vi "Dashboard Main.vi"() -> ()   [LabVIEW 2013]
uses:
  <vilib>/event_ctls.llb/eventvkey.ctl
  <vilib>/Rock Robotics/WPI/Dashboard/WPI_DashboardLogging Global.vi
  <vilib>/Utility/config.llb/Write Key (String).vi
  <vilib>/Utility/config.llb/Write Key (I32).vi
  <vilib>/Utility/config.llb/NI_LVConfig.lvlib
panel:
  out "Image Message":string="Timeout in Camera Communications"
  in  "Rec Mode":enum32{"Stop", "Record", "Playback"}(radio)
  in  "Dashboard Tab":T1(tab)
  out "Ultrasonic Sensor":dbl
  in  "Camera Settings":T2={"Frame Rate"=30, "Compression"=30, "Size"=1} {"Frame Rate" scale=1.0..30.0; "Size" items=["640x480", "320x240", "160x120"]}
  out "MotorSliders R":cluster{"MotorSlide1":dbl, "MotorSlide2":dbl} {"MotorSlide2" scale=-1.0..1.0 scale format="%#_2e"; "MotorSlide1" scale=-1.0..1.0 scale format="%#_2e"}
  out "MotorChart R":cluster{"Numeric":dbl, "Numeric":dbl}(graph)
  out "MotorSliders L":T3 {"MotorSlide4 2" scale=0.0..14.0 scale format="%#_2e"; "MotorSlide2" scale=-1.0..1.0 scale format="%#_2e"; "MotorSlide1" scale=-1.0..1.0 scale format="%#_2e"}
  out "MotorChart L":T4(graph)
  out "JS1 Z":dbl(slide) scale=-1.0..1.0 scale format="%#_2e"
  out "Joystick 1":cluster{"X":dbl, "Y":dbl}[](graph)
  out "JS Buttons 1":T5
  out "JS2 Z":dbl(slide) scale=-1.0..1.0 scale format="%#_2e"
  out "Joystick 2":cluster{"X":dbl, "Y":dbl}[](graph)
  out "JS Buttons 2":T5
  out "Mode":T6(ring)=enum."Auto Disabled"
  out "Camera IP":string
  in  "DB Camera Config":bool
  out "fps":dbl format="%#.1g"
  out "Mbps":dbl format="%#.1g"
  out "Mbps 2":bool
  out "LED 1":bool
  out "String POT":dbl
  in  "Slider 1":dbl(slide) scale=0.0..100.0
  in  "Checkbox 2":bool
  in  "Checkbox 1":bool
  in  "Test Slider":dbl(slide) scale=0.0..100.0 scale format="%#_3g"
  in  "On/Off":bool caption="Solenoid"
  in  "Test Name":u16(ring) items=["Select the test to run...", "Example Test", "-------------------------------", "List of tests is built in robot code.", "Replace with your own automated tests."]
  in  "Test Tree":string(tree)
  in  "Motor":cluster{"Value":dbl, "Enable":bool} {"Value" scale=-1.0..1.0 scale format="%#_3g"}
  out "Progress":T7 {"Test Progress" scale=0.0..100.0}
  in  "Rev/Fwd":cluster{"Forward":bool, "Reverse":bool}
  in  "Test Ring":u16(ring) items=["Auto", "Fixed indoor", "Fixed outdoor 1", "Fixed outdoor 2", "Fixed fluorescent 1", "Fixed fluorescent 2", "Hold current"]
  in  "Listbox":i32(listbox)
  out "Tree":string(tree)
  out "Camera Image":T8(plugin-control)
  in  "Enable":bool
  # "Left"
  # "Front"
  # "Right"
  # "Battery"
  # "Customize by placing controls and indicators here and name to\nmatch Dashboard Variables on robot."
  # "This tab is a great place for autonomous settings and validation.\nCustomize by placing controls and indicators here and name to\nmatch Dashboard Variables on robot."
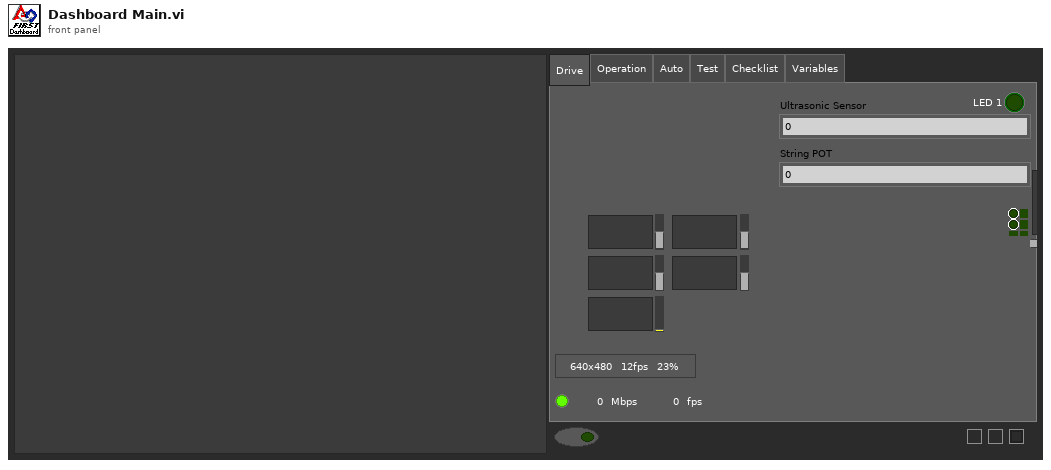
[diagram p1: front panel]
types:
  T1 = enum32{"Drive", "Operation", "Auto", "Test", "Checklist", "Variables"}
  T2 = cluster{"Frame Rate":i32, "Compression":i32, "Size":u16}
  T3 = cluster{"MotorSlide1":dbl, "MotorSlide2":dbl, "MotorSlide4 2":dbl}
  T4 = cluster{"Numeric":dbl, "Numeric":dbl, "Battery":sgl}
  T5 = cluster{bool, bool, bool, bool, bool, bool, bool, bool, bool, bool, bool, bool}
  T6 = enum8{"Tele-Op Disabled", "Tele-Op Enabled", "Auto Disabled", "Auto Enabled", "Test Disabled", "Test Enabled", ""}
  T7 = cluster{"Test Progress":u8, "Test Progress Text":string}
  T8 = typedef "IMAQ Image.ctl" = refnum<image>
  T9 = typedef "Image Type" = u32
  T10 = cluster{"Digital Inputs":bool[], "Digital Outputs":bool[]}
  T11 = cluster{"Competition mode":bool, "Robot Link":bool, "Autonomous":bool, "Enabled":bool, "E-Stop":bool, "Simulated":bool, "TestMode":bool, "Docked Window":bool}
  T12 = cluster{"Boolean Array[0]":bool, "Boolean Array[1]":bool, "Boolean Array[2]":bool, "Boolean Array[3]":bool, "Boolean Array[4]":bool, "Boolean Array[5]":bool, "Boolean Array[6]":bool, "Boolean Array[7]":bool, "Boolean Array[8]":bool, "Boolean Array[9]":bool, "Boolean Array[10]":bool, "Boolean Array[11]":bool}
  T13 = typedef "NI_LVConfig.lvlib/Config Data RefNum.ctl" = refnum<k1>
  T14 = typedef "eventvkey.ctl" = enum16{"ASCII", "Enter", "Return", "Shift", "Ctrl", "Alt", "Cmd", "Opt", "Caps", "NumLock", "Clear", "Break", "Up", "Down", "Left", "Right", "Insert", "Delete", "Home", "End", "PageUp", "PageDown", "Escape", "Help", "Pause", "ScrollLock", "F1", "F2", "F3", "F4", "F5", "F6", "F7", "F8", "F9", "F10", "F11", "F12", "F13", "F14", "F15", "F16", "F17", "F18", "F19", "F20", "F21", "F22", "F23", "F24", "Play", "VolumeUp", "VolumeDown", "Mute", "Two Byte Char"}
  T15 = cluster{"Image Size":bool, "Image Type":bool, "Pixel Value":bool, "ROI Information":bool, "Zoom Factor":bool}
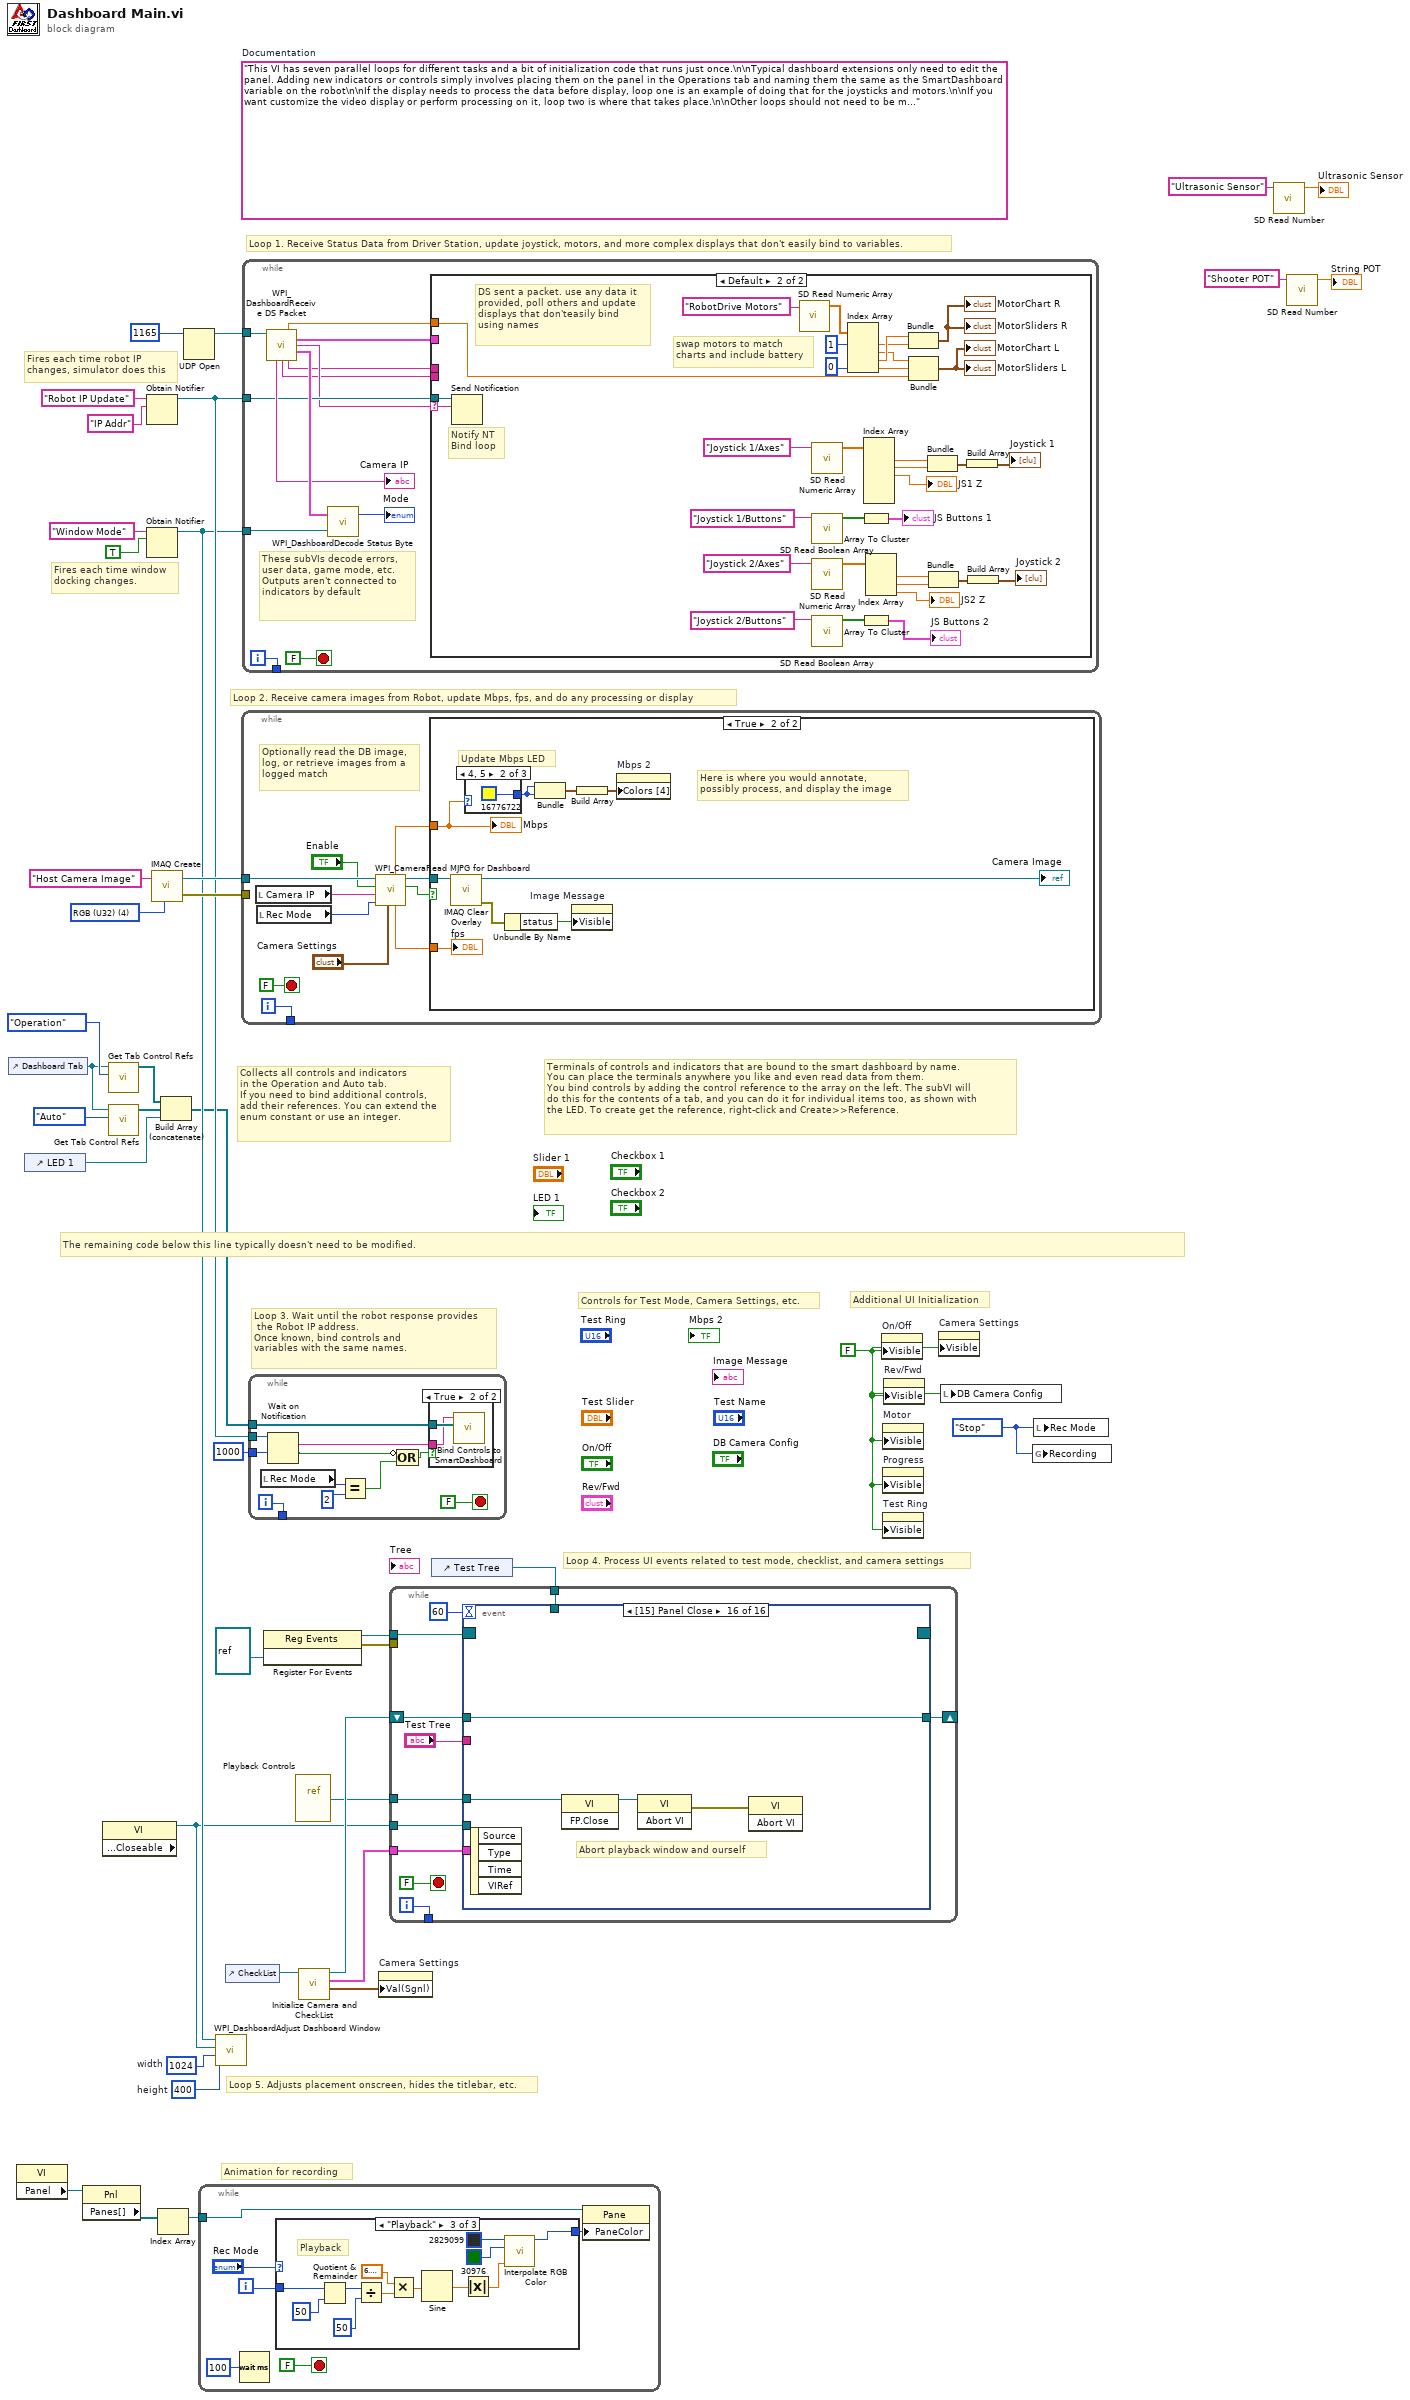
[diagram p0: block diagram]
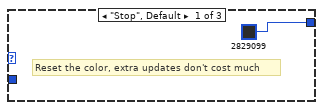
[diagram p2: hidden frame]
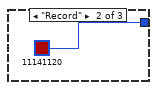
[diagram p3: hidden frame]
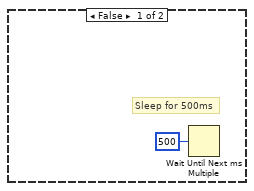
[diagram p5: hidden frame]
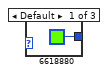
[diagram p6: hidden frame]
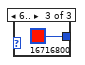
[diagram p7: hidden frame]
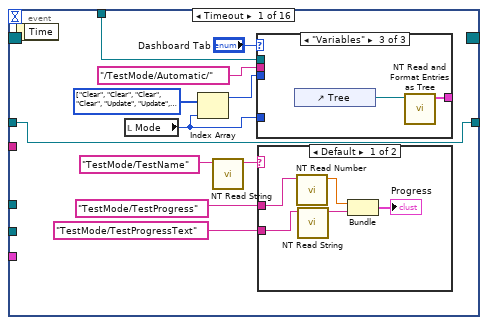
[diagram p8: hidden frame]
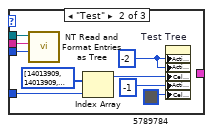
[diagram p10: hidden frame]
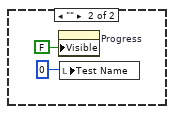
[diagram p11: hidden frame]
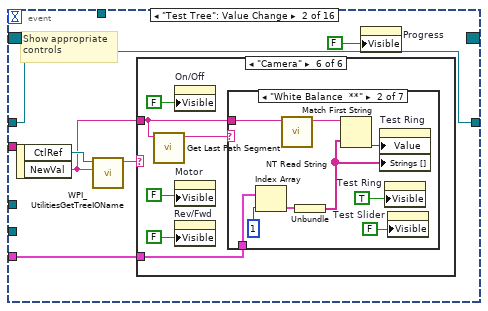
[diagram p12: hidden frame]
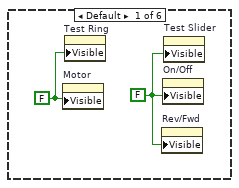
[diagram p13: hidden frame]
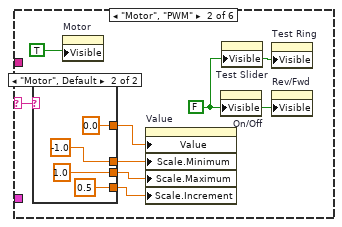
[diagram p14: hidden frame]
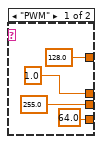
[diagram p15: hidden frame]
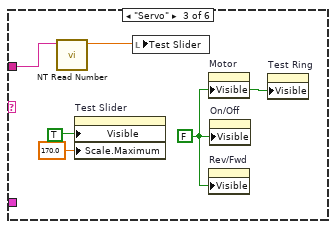
[diagram p16: hidden frame]
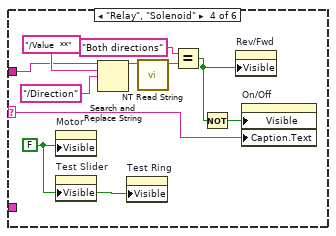
[diagram p17: hidden frame]
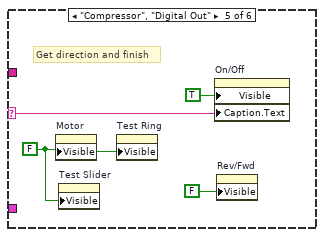
[diagram p18: hidden frame]
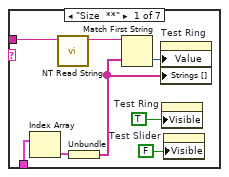
[diagram p19: hidden frame]
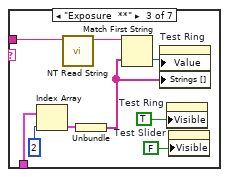
[diagram p20: hidden frame]
diagram:
  w12 = enum32{"Stop", "Record", "Playback"}."Stop" ("Rec Mode")
  w15 = 400  # height
  w16 = 1024  # width
  w29 = FALSE ("Visible")
  (unwired) "This VI has seven parallel loops for different tasks and a bit of initialization code that runs just once.\n\nTypical dashboard extensions only need to edit the panel. Adding new indicators or controls simply involves placing them on the panel in the Operations tab and naming them the same as the SmartDashboard variable on the robot\n\nIf the display needs to process the data before display, loop one is an example of doing that for the joysticks and motors.\n\nIf you want customize the video display or perform processing on it, loop two is where that takes place.\n\nOther loops should not need to be modified. They are pretty standard, and document the task they perform."  # Documentation
  w39 = T9 4 items=["Grayscale (U8)", "Grayscale (I16)", "Grayscale (SGL)", "Complex (CSG)", "RGB (U32)", "HSL (U32)", "RGB (U64)"] ("Image Type")
  # "Controls for Test Mode, Camera Settings, etc."
  # "Additional UI Initialization"
  # "Animation for recording"
  # "Fires each time robot IP\nchanges, simulator does this"
  # "Fires each time window\ndocking changes."
  # "Collects all controls and indicators\nin the Operation and Auto tab.\nIf you need to bind additional controls,\nadd their references. You can extend the\nenum constant or use an integer."
  # "The remaining code below this line typically doesn't need to be modified."
  # "Loop 4. Process UI events related to test mode, checklist, and camera settings"
  # "Terminals of controls and indicators that are bound to the smart dashboard by name.\nYou can place the terminals anywhere you like and even read data from them.\nYou bind controls by adding the control reference to the array on the left. The subVI will\ndo this for the contents of a tab, and you can do it for individual items too, as shown with\nthe LED. To create get the reference, right-click and Create>>Reference."
  # "Loop 3. Wait until the robot response provides\n the Robot IP address.\nOnce known, bind controls and\nvariables with the same names."
  # "Loop 5. Adjusts placement onscreen, hides the titlebar, etc."
  # "Loop 1. Receive Status Data from Driver Station, update joystick, motors, and more complex displays that don't easily bind to variables."
  # "Loop 2. Receive camera images from Robot, update Mbps, fps, and do any processing or display"
  n1 = control-ref of="Dashboard Tab"() -> (w10:refnum<vi>)
  n2 = property class="VI"() -> ("Panel"=w23:refnum<vi>)  [unwired: 2 in, 2 out]
  n3 = control-ref of="LED 1"() -> (w5:refnum<vi>)
  n4 = property class="Pnl"(reference=w23) -> ("Panes[]"=w24:refnum<vi>[])  [unwired: 1 in, 2 out]
  n5 = property class="VI" props=["Front Panel.Closeable"]() -> (reference out=w11:refnum<vi>)  [unwired: 2 in, 2 out]
  n6 = call <vilib>:"Get Tab Control Refs.vi"("Page Index"=T1."Operation" ("Dashboard Tab"), "TabControl in"=w10) -> ("ControlsOnPage"=w8:refnum<vi>[])  [unwired: 9 in]
  n7 = call <vilib>:"Get Tab Control Refs.vi"("Page Index"=T1."Auto" ("Dashboard Tab"), "TabControl in"=w10) -> ("ControlsOnPage"=w9:refnum<vi>[])  [unwired: 9 in]
  n8 = Obtain Notifier(name (unnamed)="Robot IP Update", notification data type="IP Addr" ("name (unnamed)")) -> (notifier out=w33:refnum<notifier>)  [unwired: 2 in, 2 out]
  n9 = Obtain Notifier(name (unnamed)="Window Mode", notification data type=TRUE) -> (notifier out=w14:refnum<notifier>)  [unwired: 2 in, 2 out]
  n10 = call "IMAQ Create"("Image Name"="Host Camera Image", "Image Type"=w39) -> ("New Image"=w37:T8, "error out"=w36:errorcluster)  [unwired: 2 in, 1 out]
  n11 = Index Array(array=w24) -> (element=w22:refnum<vi>)  [unwired: 1 in]
  n12 = Build Array (concatenate)(w8, w9, w5) -> (w7:refnum<vi>[])
  n13 = UDP Open(11:u16 1165 ("port")) -> (port=w40:refnum<k16>)  [unwired: 2 in, 4 out]
  n14 = while {
    tunnel: w22 -> [w43]
    i -> [w46]
    stop <- FALSE stop-if-true
    n15 = Wait (ms)(milliseconds to wait=u32 100) -> ()  [unwired: 1 out]
    n16 = case shown="\"Playback\"" "Rec Mode" {
      tunnel: w46 -> [_ _ w61]
      tunnel: [u32 2829099 ("Base Color") u32 11141120 ("Target Color") w50] -> w42
      frame "Stop", Default {
        # "Reset the color, extra updates don't cost much"
      }
      frame "Record" {
      }
      frame "Playback" {
        # "Playback"
        n17 = Quotient & Remainder(x=w61, y=u32 50 ("milliseconds to wait")) -> (x-y*floor(x/y)=w57:u32)  [unwired: 1 out]
        n18 = Divide(x=w57, y=u32 50 ("milliseconds to wait")) -> (x/y=w54:dbl)
        n19 = Multiply(x=6.283185307179586, y=w54) -> (x*y=w59:dbl)
        n20 = Sine(x=w59) -> (sin(x)=w58:dbl)
        n21 = Absolute Value(x=w58) -> (abs(x)=w51:dbl)
        n22 = call "Interpolate RGB Color.vi"("Proportion"=w51, "Target Color"=u32 30976, "Base Color"=u32 2829099) -> ("Result Color"=w50:u32)  [unwired: 8 in]
      }
    }
    n23 = property class="Pane"(reference=w43, "PaneColor"=w42) -> ()  [unwired: 1 in, 2 out]
  }
  n24 = call <vilib>:"WPI_DashboardAdjust Dashboard Window.vi"("height"=w15, "width"=w16, "reference in"=w11, "Notifier in"=w14) -> ()  [unwired: 8 in]
  n25 = control-ref of="CheckList"() -> (w13:refnum<vi>)
  n26 = while {
    tunnel: w37 -> [w70]
    tunnel: w36 -> [_]
    tunnel: [w71] -> _
    i -> [w71]
    stop <- FALSE stop-if-true
    # "Optionally read the DB image,\nlog, or retrieve images from a\nlogged match"
    n27 = local read "Camera IP"() -> (w63:string)
    n28 = local read "Rec Mode"() -> (w62:enum32{"Stop", "Record", "Playback"})
    n29 = call <vilib>:"WPI_CameraRead MJPG for Dashboard.vi"("Camera Settings"="Camera Settings", "Rec Mode"=w62, "Camera IP"=w63, "Enable"="Enable", "Refnum in"=w70) -> ("Active"=w67:bool, "Refnum out"=w69:T8, "FPS"=w66:dbl, "Bandwidth (Mbps)"=w65:dbl)  [unwired: 3 in]
    n30 = case shown="True" w67 {
      tunnel: w69 -> [_ w77]
      tunnel: w65 -> [_ w76]
      tunnel: w66 -> [_ w74]
      frame False {
        # "Sleep for 500ms"
        n31 = Wait Until Next ms Multiple(millisecond multiple=u32 500) -> ()  [unwired: 1 out]
      }
      frame True {
        # "Here is where you would annotate,\npossibly process, and display the image"
        # "Update Mbps LED"
        n32 = call "IMAQ Clear Overlay"("Image"=w77) -> ("error out"=w81:errorcluster, "Image Out"=→"Camera Image":T8)  [unwired: 2 in, 7 out]
        n33 = case shown="4, 5" w76 {
          tunnel: [u32 6618880 ("Color Box") u32 16776722 ("Color Box") u32 16716800 ("Color Box")] -> w78
          frame Default {
          }
          frame 4, 5 {
          }
          frame 6.. {
          }
        }
        n34 = Unbundle By Name(w81) -> ("status"=w82:bool)
        n35 = Bundle("Color Box"=w78, "Color Box"=w78) -> (w80:cluster{"Color Box":u32, "Color Box":u32})  [unwired: 1 out]
        n36 = property on="Image Message" class="Str"("Visible"=w82) -> ()  [unwired: 2 in, 2 out]
        n37 = Build Array(w80) -> (w79:cluster{"Color Box":u32, "Color Box":u32}[])
        n38 = property on="Mbps 2" class="Bool (strict)"("Colors [4]"=w79) -> ()  [unwired: 2 in, 2 out]
        "Mbps" <- w76
        "fps" <- w74
      }
    }
  }
  n39 = while {
    tunnel: w40 -> [w96]
    tunnel: w33 -> [w91]
    tunnel: w14 -> [w95]
    tunnel: [w92] -> _
    i -> [w92]
    stop <- FALSE stop-if-true
    # "These subVIs decode errors, user data, game mode, etc.\nOutputs aren't connected to indicators by default"
    n40 = call <vilib>:"WPI_DashboardReceive DS Packet.vi"("Recv Socket"=w96) -> ("Battery"=w86:sgl, "Driver Station"=w87:T10, "Robot IP Address"=w90:string, "Status"=w97:T11, "Camera IP Address"=→"Camera IP":string, "Low Priority User Data"=w89:string, "High Priority User Data"=w88:string)  [unwired: 1 in, 7 out]
    n41 = call <vilib>:"WPI_DashboardDecode Status Byte.vi"("Window Mode Notifier"=w95, "Status"=w97) -> ("Mode"=→"Mode":T6)  [unwired: 1 out]
    n42 = case shown="Default" w90 {
      selector: w90 -> [_ w109]
      tunnel: w91 -> [_ w110]
      tunnel: w89 -> [_ _]
      tunnel: w88 -> [_ _]
      tunnel: w87 -> [_ _]
      tunnel: w86 -> [_ w108]
      frame "0.0.0.0" {
        # "DS not sending packets, or no robot exists yet.\nDon't poll the variables"
      }
      frame Default {
        # "Notify NT\nBind loop"
        # "DS sent a packet. use any data it\nprovided, poll others and update\ndisplays that don'teasily bind\nusing names"
        # "swap motors to match\ncharts and include battery"
        n43 = Send Notification(notification=w109, notifier=w110) -> ()  [unwired: 1 in, 2 out]
        n44 = call <vilib>:"SD Read Numeric Array.vi"("Name"="RobotDrive Motors") -> ("Numeric Array"=w107:dbl[])  [unwired: 8 in, 2 out]
        n45 = call <vilib>:"SD Read Numeric Array.vi"("Name"="Joystick 1/Axes") -> ("Numeric Array"=w126:dbl[])  [unwired: 8 in, 2 out]
        n46 = call <vilib>:"SD Read Boolean Array.vi"("Name"="Joystick 1/Buttons") -> ("Boolean Array"=w128:bool[])  [unwired: 8 in, 2 out]
        n47 = call <vilib>:"SD Read Numeric Array.vi"("Name"="Joystick 2/Axes") -> ("Numeric Array"=w120:dbl[])  [unwired: 8 in, 2 out]
        n48 = call <vilib>:"SD Read Boolean Array.vi"("Name"="Joystick 2/Buttons") -> ("Boolean Array"=w119:bool[])  [unwired: 8 in, 2 out]
        n49 = Index Array(array=w107, index #1=1, index #4=0) -> (element #1=w103:dbl, element #2=w102:dbl, element #3=w104:dbl, element #4=w99:dbl)  [unwired: 2 in]
        n50 = Array To Cluster(array=w128) -> (cluster=→"JS Buttons 1":T12)
        n51 = Array To Cluster(array=w119) -> (cluster=→"JS Buttons 2":T12)
        n52 = Index Array(array=w126) -> (element #1=w123:dbl, element #2=w124:dbl, element #3=→"JS1 Z":dbl)  [unwired: 6 in, 3 out]
        n53 = Index Array(array=w120) -> (element #1=w115:dbl, element #2=w114:dbl, element #3=→"JS2 Z":dbl)  [unwired: 3 in]
        n54 = Bundle("Numeric"=w104, "Numeric"=w103) -> (→"MotorChart R" →"MotorSliders R":cluster{"Numeric":dbl, "Numeric":dbl})  [unwired: 1 in]
        n55 = Bundle("Numeric"=w102, "Numeric"=w99, "Battery"=w108) -> (→"MotorChart L" →"MotorSliders L":T4)  [unwired: 1 in]
        n56 = Bundle("Numeric"=w123, "Numeric"=w124) -> (w122:cluster{"Numeric":dbl, "Numeric":dbl})  [unwired: 1 in]
        n57 = Bundle("Numeric"=w115, "Numeric"=w114) -> (w116:cluster{"Numeric":dbl, "Numeric":dbl})  [unwired: 1 in]
        n58 = Build Array(w122) -> (→"Joystick 1":cluster{"Numeric":dbl, "Numeric":dbl}[])
        n59 = Build Array(w116) -> (→"Joystick 2":cluster{"Numeric":dbl, "Numeric":dbl}[])
      }
    }
  }
  n60 = while {
    tunnel: w7 -> [w142]
    tunnel: w33 -> [w140]
    tunnel: [w138] -> _
    tunnel: u32 1000 ("milliseconds to wait") -> [w137]
    i -> [w138]
    stop <- FALSE stop-if-true
    n61 = local read "Rec Mode"() -> (w133:enum32{"Stop", "Record", "Playback"})
    n62 = Wait on Notification(notifier=w140, timeout in ms (-1)=w137) -> (notification=w139:string, timed out?=w135:bool)  [unwired: 2 in, 2 out]
    n63 = Equal?(x=w133, y=u16 2 ("Rec Mode")) -> (x = y?=w134:bool)
    n64 = Compound Arithmetic op=OR(invert w135, w134) -> (w136:bool)
    n65 = case shown="True" w136 {
      tunnel: w142 -> [_ w144]
      tunnel: w139 -> [_ w143]
      frame False {
      }
      frame True {
        n66 = call <vilib>:"Bind Controls to SmartDashboard.vi"("Bound Control Refs"=w144, "Server IP Address"=w143) -> ()  [unwired: 10 in]
      }
    }
  }
  n67 = register-events(refnum<vi> refnum) -> (reference out=w20:refnum<event-registration>, error out=w19:errorcluster)  [unwired: 2 in]
  n68 = vi-ref "Playback Controls.vi"() -> (w21:refnum<vi>)
  n69 = call "Initialize Camera and CheckList.vi"("ListBox in"=w13) -> ("Cluster"=w27:cluster{"value":i32, "value":i32, "index":i32}, "Array"=w28:cluster{string[]}[], "File Refnum"=w26:T13)  [unwired: 8 in]
  n70 = property on="Camera Settings" class="Clust (strict)"("Val(Sgnl)"=w27) -> ()  [unwired: 2 in, 2 out]
  n71 = control-ref of="Test Tree"() -> (w25:refnum<vi>)
  n72 = while {
    tunnel: w28 -> [w152]
    shift-right: [w151] -> _
    shift-left: w26 -> [w150]
    tunnel: [w149] -> _
    tunnel: w25 -> [w148]
    tunnel: w21 -> [w147]
    tunnel: w20 -> [w146]
    tunnel: w19 -> [_]
    tunnel: w11 -> [w145]
    i -> [w149]
    stop <- FALSE stop-if-true
    n73 = event shown="[15] Panel Close" {
      selector: w146 -> [_ _ _ _ _ _ _ _ _ _ _ _ _ _ _ _]
      dyn-events: [_ _ _ _ _ _ _ _ _ _ _ _ _ w390 _ _] -> _
      timeout: u32 60 ("milliseconds to wait") -> [_ _ _ _ _ _ _ _ _ _ _ _ _ _ _ _]
      tunnel: w148 -> [w162 _ _ _ _ _ _ _ _ _ _ _ _ _ _ _]
      tunnel: "Test Tree" -> [_ _ _ _ _ _ _ _ w359 w367 w369 w373 w381 _ _ _]
      tunnel: w152 -> [_ w186 _ _ _ _ w323 w353 _ _ _ _ _ _ _ _]
      tunnel: [w156 w185 w284 w289 w297 w309 w322 w346 w358 w365 w368 w372 w380 w392 w406 w407] -> w151
      tunnel: w150 -> [w156 w185 w284 w289 w297 w309 w321 w346 w358 w365 w368 w372 w380 w392 w406 w407]
      tunnel: w147 -> [_ _ _ _ _ _ _ _ _ _ _ _ _ w393 _ w410]
      tunnel: w145 -> [_ _ _ _ _ _ _ _ _ _ _ _ _ w388 _ _]
      event Timeout {
        w161 = enum16{"Update", "Clear"}[] [enum."Clear", enum."Clear", enum."Clear", enum."Clear", enum."Update", enum."Update", enum."Clear"] items=["Update", "Clear"]
        n74 = event-data() -> ()  [unwired: 1 in, 1 out]
        n75 = local read "Mode"() -> (w159:T6)
        n76 = Index Array(array=w161, index=w159) -> (element=w160:enum16{"Update", "Clear"})
        n77 = call <vilib>:"NT Read String.vi"("Name"="TestMode/TestName") -> ("String"=w165:string)  [unwired: 9 in, 1 out]
        n78 = case shown="\"Variables\"" "Dashboard Tab" {
          tunnel: w162 -> [_ w175 _]
          tunnel: "/TestMode/Automatic/" ("Name Pattern") -> [_ w174 _]
          tunnel: w160 -> [_ w173 _]
          tunnel: w159 -> [_ w171 _]
          tunnel: [_ _ w177] -> _
          frame "Operation", Default {
          }
          frame "Test" {
            w170 = -2 ("Active Item:Row Number")
            n79 = call <vilib>:"NT Read and Format Entries as Tree.vi"("Operation"=w173, "Name Pattern"=w174, "Tree Refnum"=w175) -> ()  [unwired: 7 in, 2 out]
            n80 = Index Array(array=u32[] [14013909, 14013909, 14013909, 14013909, 14013909, 16777215, 14013909], index=w171) -> (element=w169:u32)
            n81 = property on="Test Tree" class="Tree (strict)"("Active Item Row Number"=w170, "ActiveColNum"=w170, "CellBG"=w169, "Active Item Row Number"=-1 ("Active Item:Row Number"), "CellBG"=u32 5789784 ("Color Box")) -> ()  [unwired: 2 in, 2 out]
          }
          frame "Variables" {
            n82 = control-ref of="Tree"() -> (w176:refnum<vi>)
            n83 = call <vilib>:"NT Read and Format Entries as Tree.vi"("Tree Refnum"=w176) -> ("Formatted Strings"=w177:cluster{"Name":string, "Value":string}[])  [unwired: 9 in, 1 out]
          }
        }
        n84 = case shown="Default" w165 {
          tunnel: "TestMode/TestProgress" ("Name") -> [w179 _]
          tunnel: "TestMode/TestProgressText" ("Name") -> [w178 _]
          frame Default {
            n85 = call <vilib>:"NT Read Number.vi"("Name"=w179) -> ("Numeric"=w180:dbl)  [unwired: 9 in, 1 out]
            n86 = call <vilib>:"NT Read String.vi"("Name"=w178) -> ("String"=w181:string)  [unwired: 9 in, 1 out]
            n87 = Bundle("Numeric"=w180, "String"=w181) -> (→"Progress":cluster{"Numeric":dbl, "String":string})  [unwired: 1 in]
          }
          frame "" {
            n88 = property on="Progress" class="Clust (strict)"("Visible"=FALSE) -> ()  [unwired: 2 in, 2 out]
            n89 = local write "Test Name"(u16 0) -> ()
          }
        }
      }
      event "Test Tree": Value Change {
        # "Show appropriate\ncontrols"
        n90 = event-data() -> ("CtlRef"=w189:refnum<vi>, "NewVal"=w187:string)  [unwired: 1 in]
        n91 = call <vilib>:"WPI_UtilitiesGetTreeIOName.vi"("NewVal"=w187, "TreeControl in"=w189) -> ("I/O Name"=w190:string)  [unwired: 9 in]
        n92 = case shown="\"Camera\"" w190 {
          selector: w190 -> [_ w197 _ w215 w224 _]
          tunnel: w187 -> [_ _ w212 w214 _ w231]
          tunnel: w186 -> [_ _ _ _ _ w230]
          frame Default {
            w192 = FALSE ("Visible")
            w191 = FALSE ("Visible")
            n93 = property on="Motor" class="Clust (strict)"("Visible"=w191) -> ()  [unwired: 2 in, 2 out]
            n94 = property on="Test Ring" class="Ring (strict)"("Visible"=w191) -> ()  [unwired: 2 in, 2 out]
            n95 = property on="Rev/Fwd" class="Clust (strict)"("Visible"=w192) -> ()  [unwired: 2 in, 2 out]
            n96 = property on="On/Off" class="Bool (strict)"("Visible"=w192) -> ()  [unwired: 2 in, 2 out]
            n97 = property on="Test Slider" class="Slide (strict)"("Visible"=w192) -> ()  [unwired: 2 in, 2 out]
          }
          frame "Motor", "PWM" {
            w198 = FALSE ("Visible")
            n98 = case shown="\"Motor\", Default" w197 {
              tunnel: [1.0 ("Value") -1.0 ("Value")] -> w196
              tunnel: [255.0 ("Value") 1.0 ("Value")] -> w195
              tunnel: [128.0 ("Value") 0.0 ("Value")] -> w194
              tunnel: [64.0 ("Value") 0.5 ("Value")] -> w193
              frame "PWM" {
              }
              frame "Motor", Default {
              }
            }
            n99 = property on="Motor" class="Clust (strict)"("Visible"=TRUE) -> ()  [unwired: 2 in, 2 out]
            n100 = property on="Value" class="Slide (strict)"("Value"=w194, "Scale.Minimum"=w196, "Scale.Maximum"=w195, "Scale.Increment"=w193) -> ()  [unwired: 2 in, 2 out]
            n101 = property on="On/Off" class="Bool (strict)"("Visible"=w198) -> ()  [unwired: 2 in, 2 out]
            n102 = property on="Test Slider" class="Slide (strict)"("Visible"=w198) -> ()  [unwired: 2 in, 2 out]
            n103 = property on="Test Ring" class="Ring (strict)"("Visible"=w198) -> ()  [unwired: 2 in, 2 out]
            n104 = property on="Rev/Fwd" class="Clust (strict)"("Visible"=w198) -> ()  [unwired: 2 in, 2 out]
          }
          frame "Servo" {
            w210 = FALSE ("Visible")
            n105 = call <vilib>:"NT Read Number.vi"("Name"=w212) -> ("Numeric"=w211:dbl)  [unwired: 9 in, 1 out]
            n106 = property on="Test Slider" class="Slide (strict)"("Visible"=TRUE, "Scale.Maximum"=170.0 ("Scale.Range:Maximum")) -> ()  [unwired: 2 in, 2 out]
            n107 = local write "Test Slider"(w211) -> ()
            n108 = property on="Motor" class="Clust (strict)"("Visible"=w210) -> ()  [unwired: 2 in, 2 out]
            n109 = property on="Rev/Fwd" class="Clust (strict)"("Visible"=w210) -> ()  [unwired: 2 in, 2 out]
            n110 = property on="On/Off" class="Bool (strict)"("Visible"=w210) -> ()  [unwired: 2 in, 2 out]
            n111 = property on="Test Ring" class="Ring (strict)"("Visible"=w210) -> ()  [unwired: 2 in, 2 out]
          }
          frame "Relay", "Solenoid" {
            w213 = FALSE ("Visible")
            n112 = property on="Motor" class="Clust (strict)"("Visible"=w213) -> ()  [unwired: 2 in, 2 out]
            n113 = property on="Test Slider" class="Slide (strict)"("Visible"=w213) -> ()  [unwired: 2 in, 2 out]
            n114 = Search and Replace String(input string=w214, search string="/Value  **", replace string="/Direction") -> (result string=w220:string)  [unwired: 5 in, 3 out]
            n115 = property on="Test Ring" class="Ring (strict)"("Visible"=w213) -> ()  [unwired: 2 in, 2 out]
            n116 = call <vilib>:"NT Read String.vi"("Name"=w220) -> ("String"=w218:string)  [unwired: 9 in, 1 out]
            n117 = Equal?(x="Both directions", y=w218) -> (x = y?=w216:bool)
            n118 = Not(x=w216) -> (.not. x?=w217:bool)
            n119 = property on="Rev/Fwd" class="Clust (strict)"("Visible"=w216) -> ()  [unwired: 2 in, 2 out]
            n120 = property on="On/Off" class="Bool (strict)"("Visible"=w217, "Caption.Text"=w215) -> ()  [unwired: 2 in, 2 out]
          }
          frame "Compressor", "Digital Out" {
            w223 = FALSE ("Visible")
            # "Get direction and finish"
            n121 = property on="Motor" class="Clust (strict)"("Visible"=w223) -> ()  [unwired: 2 in, 2 out]
            n122 = property on="Test Slider" class="Slide (strict)"("Visible"=w223) -> ()  [unwired: 2 in, 2 out]
            n123 = property on="Test Ring" class="Ring (strict)"("Visible"=w223) -> ()  [unwired: 2 in, 2 out]
            n124 = property on="On/Off" class="Bool (strict)"("Visible"=TRUE, "Caption.Text"=w224) -> ()  [unwired: 2 in, 2 out]
            n125 = property on="Rev/Fwd" class="Clust (strict)"("Visible"=FALSE) -> ()  [unwired: 2 in, 2 out]
          }
          frame "Camera" {
            n126 = call <vilib>:"Get Last Path Segment.vi"("String in"=w231) -> ("String out"=w232:string)  [unwired: 10 in]
            n127 = property on="On/Off" class="Bool (strict)"("Visible"=FALSE) -> ()  [unwired: 2 in, 2 out]
            n128 = property on="Motor" class="Clust (strict)"("Visible"=FALSE) -> ()  [unwired: 2 in, 2 out]
            n129 = property on="Rev/Fwd" class="Clust (strict)"("Visible"=FALSE) -> ()  [unwired: 2 in, 2 out]
            n130 = case shown="\"White Balance  **\"" w232 {
              tunnel: w231 -> [w238 w247 w256 w265 w274 _ w280]
              tunnel: w230 -> [w236 w244 w253 w262 w271 _ _]
              frame "Size  **" {
                n131 = Index Array(array=w236) -> (element=w235:cluster{string[]})  [unwired: 1 in]
                n132 = call <vilib>:"NT Read String.vi"("Name"=w238) -> ("String"=w237:string)  [unwired: 9 in, 1 out]
                n133 = Unbundle(w235) -> (w233:string[])
                n134 = Match First String(2:w233, 3:w237) -> (0:w234:i32)  [unwired: 1 out]
                n135 = property on="Test Ring" class="Ring (strict)"("Value"=w234, "Strings []"=w233) -> ()  [unwired: 2 in, 2 out]
                n136 = property on="Test Ring" class="Ring (strict)"("Visible"=TRUE) -> ()  [unwired: 2 in, 2 out]
                n137 = property on="Test Slider" class="Slide (strict)"("Visible"=FALSE) -> ()  [unwired: 2 in, 2 out]
              }
              frame "White Balance  **" {
                n138 = Index Array(array=w244, index=1) -> (element=w245:cluster{string[]})
                n139 = call <vilib>:"NT Read String.vi"("Name"=w247) -> ("String"=w246:string)  [unwired: 9 in, 1 out]
                n140 = Unbundle(w245) -> (w242:string[])
                n141 = Match First String(2:w242, 3:w246) -> (0:w241:i32)  [unwired: 1 out]
                n142 = property on="Test Ring" class="Ring (strict)"("Value"=w241, "Strings []"=w242) -> ()  [unwired: 2 in, 2 out]
                n143 = property on="Test Ring" class="Ring (strict)"("Visible"=TRUE) -> ()  [unwired: 2 in, 2 out]
                n144 = property on="Test Slider" class="Slide (strict)"("Visible"=FALSE) -> ()  [unwired: 2 in, 2 out]
              }
              frame "Exposure  **" {
                n145 = Index Array(array=w253, index=2) -> (element=w254:cluster{string[]})
                n146 = call <vilib>:"NT Read String.vi"("Name"=w256) -> ("String"=w255:string)  [unwired: 9 in, 1 out]
                n147 = Unbundle(w254) -> (w250:string[])
                n148 = Match First String(2:w250, 3:w255) -> (0:w251:i32)  [unwired: 1 out]
                n149 = property on="Test Ring" class="Ring (strict)"("Value"=w251, "Strings []"=w250) -> ()  [unwired: 2 in, 2 out]
                n150 = property on="Test Ring" class="Ring (strict)"("Visible"=TRUE) -> ()  [unwired: 2 in, 2 out]
                n151 = property on="Test Slider" class="Slide (strict)"("Visible"=FALSE) -> ()  [unwired: 2 in, 2 out]
              }
              frame "Exposure Priority  **" {
                n152 = Index Array(array=w262, index=3) -> (element=w263:cluster{string[]})
                n153 = call <vilib>:"NT Read String.vi"("Name"=w265) -> ("String"=w264:string)  [unwired: 9 in, 1 out]
                n154 = Unbundle(w263) -> (w259:string[])
                n155 = Match First String(2:w259, 3:w264) -> (0:w260:i32)  [unwired: 1 out]
                n156 = property on="Test Ring" class="Ring (strict)"("Value"=w260, "Strings []"=w259) -> ()  [unwired: 2 in, 2 out]
                n157 = property on="Test Ring" class="Ring (strict)"("Visible"=TRUE) -> ()  [unwired: 2 in, 2 out]
                n158 = property on="Test Slider" class="Slide (strict)"("Visible"=FALSE) -> ()  [unwired: 2 in, 2 out]
              }
              frame "Color Enable  **" {
                n159 = Index Array(array=w271, index=4) -> (element=w272:cluster{string[]})
                n160 = call <vilib>:"NT Read String.vi"("Name"=w274) -> ("String"=w273:string)  [unwired: 9 in, 1 out]
                n161 = Unbundle(w272) -> (w268:string[])
                n162 = Match First String(2:w268, 3:w273) -> (0:w269:i32)  [unwired: 1 out]
                n163 = property on="Test Ring" class="Ring (strict)"("Value"=w269, "Strings []"=w268) -> ()  [unwired: 2 in, 2 out]
                n164 = property on="Test Ring" class="Ring (strict)"("Visible"=TRUE) -> ()  [unwired: 2 in, 2 out]
                n165 = property on="Test Slider" class="Slide (strict)"("Visible"=FALSE) -> ()  [unwired: 2 in, 2 out]
              }
              frame Default {
                n166 = property on="Test Ring" class="Ring (strict)"("Visible"=FALSE) -> ()  [unwired: 2 in, 2 out]
                n167 = property on="Test Slider" class="Slide (strict)"("Visible"=FALSE) -> ()  [unwired: 2 in, 2 out]
              }
              frame "Brightness  **", "Color Level  **", "Compression  **", "FPS  **", "Sharpness  **" {
                n168 = call <vilib>:"NT Read Number.vi"("Name"=w280) -> ("Numeric"=w279:dbl)  [unwired: 9 in, 1 out]
                n169 = local write "Test Slider"(w279) -> ()
                n170 = property on="Test Slider" class="Slide (strict)"("Visible"=TRUE, "Scale.Maximum"=100.0 ("Scale.Range:Maximum")) -> ()  [unwired: 2 in, 2 out]
                n171 = property on="Test Ring" class="Ring (strict)"("Visible"=FALSE) -> ()  [unwired: 2 in, 2 out]
              }
            }
          }
        }
        n172 = property on="Progress" class="Clust (strict)"("Visible"=FALSE) -> ()  [unwired: 2 in, 2 out]
      }
      event "Test Name": Mouse Enter {
        # "Populate the ring with the list of tests"
        n173 = event-data() -> ()  [unwired: 1 in, 1 out]
        n174 = call <vilib>:"NT Read String Array.vi"("Name"="TestMode/TestList") -> ("String Array"=w288:string[])  [unwired: 9 in, 1 out]
        n175 = Build Array (concatenate)("Select the test to run...", w288) -> (w287:string[])
        n176 = property on="Test Name" class="Ring (strict)"("Strings []"=w287) -> ()  [unwired: 2 in, 2 out]
      }
      event "Test Name": Value Change {
        w290 = FALSE ("Visible")
        # "Tell the robot the test name to run"
        n177 = event-data() -> ("NewVal"=w294:u16)  [unwired: 1 in]
        n178 = property on="Test Name" class="Ring (strict)"() -> ("Strings []"=w295:string[])  [unwired: 2 in, 2 out]
        n179 = local write "Progress"(T7 {"Test Progress"=0, "Test Progress Text"=""} ("Progress")) -> ()
        n180 = Index Array(array=w295, index=w294) -> (element=w293:string)
        n181 = call <vilib>:"NT Write String.vi"("String"=w293, "Name"="TestMode/TestName") -> ()  [unwired: 9 in, 1 out]
        n182 = property on="Progress" class="Clust (strict)"("Visible"=TRUE) -> ()  [unwired: 2 in, 2 out]
        n183 = property on="Motor" class="Clust (strict)"("Visible"=w290) -> ()  [unwired: 2 in, 2 out]
        n184 = property on="Test Slider" class="Slide (strict)"("Visible"=w290) -> ()  [unwired: 2 in, 2 out]
        n185 = property on="On/Off" class="Bool (strict)"("Visible"=w290) -> ()  [unwired: 2 in, 2 out]
        n186 = property on="Rev/Fwd" class="Clust (strict)"("Visible"=w290) -> ()  [unwired: 2 in, 2 out]
        n187 = property on="Test Ring" class="Ring (strict)"("Visible"=w290) -> ()  [unwired: 2 in, 2 out]
      }
      event "Listbox": Double Click {
        n188 = event-data() -> ("PlatMods.Shift"=w298:bool, "Row"=w300:i32)  [unwired: 1 in]
        n189 = case shown="True" w298 {
          tunnel: w300 -> [w304 _]
          tunnel: 1 -> [w303 _]
          frame False {
            n190 = property on="Listbox" class="LstBox (strict)"() -> ("Item Symbols"=w302:i32[])  [unwired: 2 in, 2 out]
            n191 = Replace Array Subset(array=w302, new element=w303, index=w304) -> (w301:i32[])
            n192 = property on="Listbox" class="LstBox (strict)"("Item Symbols"=w301) -> ()  [unwired: 2 in, 2 out]
          }
          frame True {
            w305 = 0 ("Top Row")
            n193 = property on="Listbox" class="LstBox (strict)"() -> ("Number of Rows"=w307:u32)  [unwired: 2 in, 2 out]
            n194 = Initialize Array(0, w307) -> (w306:i32[])
            n195 = property on="Listbox" class="LstBox (strict)"("Top Row"=w305, "Value"=w305, "Item Symbols"=w306) -> ()  [unwired: 2 in, 2 out]
          }
        }
      }
      event "Listbox": Key Down {
        n196 = event-data() -> ("VKey"=w311:T14)  [unwired: 1 in]
        n197 = case shown="\"Left\", \"Right\"" w311 {
          selector: w311 -> [w316 _]
          tunnel: eventvkey."Left" ("VKey") -> [w314 _]
          frame "Left", "Right" {
            n198 = Equal?(x=w314, y=w316) -> (x = y?=w315:bool)
            n199 = Select(t=0, s=w315, f=1) -> (s? t:f=w317:i32)
            n200 = property on="Listbox" class="LstBox (strict)"() -> ("Item Symbols"=w320:i32[])  [unwired: 2 in, 2 out]
            n201 = Replace Array Subset(array=w320, new element=w317, index="Listbox") -> (w319:i32[])
            n202 = property on="Listbox" class="LstBox (strict)"("Item Symbols"=w319) -> ()  [unwired: 2 in, 2 out]
          }
          frame Default {
          }
        }
      }
      event "DB Camera Config": Value Change {
        n203 = event-data() -> ("NewVal"=w324:bool)  [unwired: 1 in]
        n204 = case shown="False" w324 {
          tunnel: w323 -> [w333 _]
          tunnel: [w326 w344] -> w322
          tunnel: w321 -> [w325 w344]
          frame False {
            w340 = "Camera"
            w343 = FALSE ("Visible")
            n205 = local read "Camera Settings"() -> (w332:T2)
            n206 = Index Array(array=w333) -> (element=w336:cluster{string[]})  [unwired: 1 in]
            n207 = Unbundle(w332) -> ("Frame Rate"=w331:i32, "Compression"=w330:i32, "Size"=w334:u16)
            n208 = Unbundle(w336) -> (w335:string[])
            n209 = Index Array(array=w335, index=w334) -> (element=w329:string)
            n210 = call-poly <vilib>:"Write Key.vi"("section"=w340, "value"=w329, "key"="Size", "refnum"=w325) -> ("refnum out"=w342:T13)  [unwired: 2 in, 5 out]
            n211 = call-poly <vilib>:"Write Key.vi"("section"=w340, "value"=w331, "key"="FrameRate", "refnum"=w342) -> ("refnum out"=w341:T13)  [unwired: 1 in, 6 out]
            n212 = property on="Camera Settings" class="Clust (strict)"("Visible"=w343) -> ()  [unwired: 2 in, 2 out]
            n213 = local write "DB Camera Config"(w343) -> ()
            n214 = call-poly <vilib>:"Write Key.vi"("section"=w340, "value"=w330, "key"="Compression", "refnum"=w341) -> ("refnum out"=w327:T13)  [unwired: 1 in, 6 out]
            n215 = call <vilib>:"Close Config Data.vi"("refnum"=w327) -> ("file path"=w328:path)  [unwired: 2 in, 8 out]
            n216 = call <vilib>:"Open Config Data.vi"("configuration file path"=w328) -> ("refnum"=w326:T13)  [unwired: 8 in, 2 out]
          }
          frame True {
            n217 = property on="Camera Settings" class="Clust (strict)"("Visible"=TRUE) -> ()  [unwired: 2 in, 2 out]
          }
        }
      }
      event "Camera Settings": Value Change {
        n218 = event-data() -> ("NewVal"=w357:T2)  [unwired: 1 in]
        n219 = Index Array(array=w353) -> (element=w352:cluster{string[]})  [unwired: 1 in]
        n220 = Unbundle(w357) -> ("Frame Rate"=w348:i32, "Compression"=w347:i32, "Size"=w350:u16)
        n221 = Unbundle(w352) -> (w351:string[])
        n222 = Index Array(array=w351, index=w350) -> (element=w349:string)
        n223 = Format Into String(format string="%s   %dfps   %d%%", w349, w348, w347) -> (resulting string=w354:string)  [unwired: 2 in, 1 out]
        n224 = Build Array(w354) -> (w355:string[])
        n225 = property on="DB Camera Config" class="Bool (strict)"("Strings [4]"=w355) -> ()  [unwired: 2 in, 2 out]
      }
      event "Motor.Enable": Value Change {
        n226 = event-data() -> ("NewVal"=w363:bool)  [unwired: 1 in]
        n227 = Unbundle("Motor") -> ("Value"=w362:dbl)  [unwired: 1 out]
        n228 = Select(t=w362, s=w363, f=0.0) -> (s? t:f=w360:dbl)
        n229 = call <vilib>:"NT Write Number.vi"("Numeric"=w360, "Name"=w359) -> ()  [unwired: 9 in, 1 out]
      }
      event "Test Slider": Value Change {
        n230 = event-data() -> ("NewVal"=w366:dbl)  [unwired: 1 in]
        n231 = call <vilib>:"NT Write Number.vi"("Numeric"=w366, "Name"=w367) -> ()  [unwired: 9 in, 1 out]
      }
      event "On/Off": Value Change {
        n232 = event-data() -> ("NewVal"=w371:bool)  [unwired: 1 in]
        n233 = Boolean To (0,1)(Boolean=w371) -> (0, 1=w370:i16)
        n234 = call <vilib>:"NT Write Number.vi"("Numeric"=w370, "Name"=w369) -> ()  [unwired: 9 in, 1 out]
      }
      event "Rev/Fwd": Value Change {
        n235 = event-data() -> ("NewVal.Forward"=w379:bool, "NewVal.Reverse"=w378:bool)  [unwired: 1 in]
        n236 = Boolean To (0,1)(Boolean=w379) -> (0, 1=w375:i16)
        n237 = Boolean To (0,1)(Boolean=w378) -> (0, 1=w377:i16)
        n238 = Negate(x=w377) -> (-x=w376:i16)
        n239 = Add(x=w375, y=w376) -> (x+y=w374:i16)
        n240 = call <vilib>:"NT Write Number.vi"("Numeric"=w374, "Name"=w373) -> ()  [unwired: 9 in, 1 out]
      }
      event "Test Ring": Value Change {
        n241 = event-data() -> ("NewVal"=w383:u16)  [unwired: 1 in]
        n242 = property on="Test Ring" class="Ring (strict)"() -> ("Strings []"=w384:string[])  [unwired: 2 in, 2 out]
        n243 = Index Array(array=w384, index=w383) -> (element=w382:string)
        n244 = call <vilib>:"NT Write String.vi"("String"=w382, "Name"=w381) -> ()  [unwired: 9 in, 1 out]
      }
      event "Rec Mode": Value Change {
        # "Update globals for recording mode and path to read log from.\nClear when logging and let NetworkTables set path for vision to\nuse."
        n245 = event-data() -> ("NewVal"=w394:enum32{"Stop", "Record", "Playback"})  [unwired: 1 in]
        n246 = global write "WPI_DashboardLogging Global.vi" "Logging Filename"(path "") -> ()
        n247 = case shown="\"Stop\", \"Record\"" w394 {
          tunnel: w393 -> [_ w396 w404]
          tunnel: [_ _ w403] -> w390
          tunnel: [_ _ w402] -> _
          tunnel: w388 -> [_ _ w400]
          tunnel: cluster{i32, i32} {-250, 170} -> [_ _ w399]
          tunnel: [_ _ T15 {"Image Size"=TRUE, "Image Type"=TRUE, "Pixel Value"=TRUE, "ROI Information"=TRUE, "Zoom Factor"=FALSE} ("Image Information Shown:All Elements")] -> w386
          tunnel: [_ _ TRUE ("Zoom Factor")] -> w385
          frame Default {
          }
          frame "Stop", "Record" {
            # "Place Window too"
            n248 = invoke class="VI" method="FP.Close"(reference=w396) -> (reference out=w395:refnum<vi>)  [unwired: 2 in, 2 out]
            n249 = invoke class="VI" method="Abort VI"(reference=w395) -> ()  [unwired: 2 in, 3 out]
          }
          frame "Playback" {
            n250 = call "Open Playback Panel.vi"("Offset"=w399, "DB VI Ref"=w400, "Playback in"=w404) -> ("Playback out"=w401:refnum<vi>)  [unwired: 8 in]
            n251 = register-events(w401) -> (reference out=w403:refnum<event-registration>, error out=w402:errorcluster)  [unwired: 2 in]
          }
        }
        n252 = global write "WPI_DashboardLogging Global.vi" "Recording"(w394) -> ()
        n253 = property on="Camera Image" class="ImageControl"("Image Information Shown"=w386, "Image Information Visible"=w385) -> ()  [unwired: 2 in, 2 out]
        n254 = call <vilib>:"WPI_DashboardNT Log FieldName Cache.vi"("Operation"=enum16{"Lookup/Add", "Index", "Clear"}."Clear") -> ()  [unwired: 8 in, 3 out]
      }
      event Panel Close {
        w405 = enum32{"Stop", "Record", "Playback"}."Stop" ("Rec Mode")
        n255 = event-data() -> ()  [unwired: 1 in, 4 out]
        n256 = local write "Rec Mode"(w405) -> ()
        n257 = global write "WPI_DashboardLogging Global.vi" "Recording"(w405) -> ()
      }
      event Panel Close {
        # "Abort playback window and ourself"
        n258 = event-data() -> ()  [unwired: 1 in, 4 out]
        n259 = invoke class="VI" method="FP.Close"(reference=w410) -> (reference out=w409:refnum<vi>)  [unwired: 2 in, 2 out]
        n260 = invoke class="VI" method="Abort VI"(reference=w409) -> (error out=w408:errorcluster)  [unwired: 2 in, 2 out]
        n261 = invoke class="VI" method="Abort VI"(error in=w408) -> ()  [unwired: 2 in, 3 out]
      }
    }
  }
  n262 = property on="On/Off" class="Bool (strict)"("Visible"=w29) -> ()  [unwired: 2 in, 2 out]
  n263 = property on="Motor" class="Clust (strict)"("Visible"=w29) -> ()  [unwired: 2 in, 2 out]
  n264 = property on="Progress" class="Clust (strict)"("Visible"=w29) -> ()  [unwired: 2 in, 2 out]
  n265 = property on="Test Ring" class="Ring (strict)"("Visible"=w29) -> ()  [unwired: 2 in, 2 out]
  n266 = property on="Rev/Fwd" class="Clust (strict)"("Visible"=w29) -> ()  [unwired: 2 in, 2 out]
  n267 = property on="Camera Settings" class="Clust (strict)"("Visible"=w29) -> ()  [unwired: 2 in, 2 out]
  n268 = local write "DB Camera Config"(w29) -> ()
  n269 = global write "WPI_DashboardLogging Global.vi" "Recording"(w12) -> ()
  n270 = local write "Rec Mode"(w12) -> ()
  n271 = call <vilib>:"SD Read Number.vi"("Name"="Ultrasonic Sensor") -> ("Numeric"=→"Ultrasonic Sensor":dbl)  [unwired: 8 in, 2 out]
  n272 = call <vilib>:"SD Read Number.vi"("Name"="Shooter POT") -> ("Numeric"=→"String POT":dbl)  [unwired: 8 in, 2 out]
